vi "TachDataGcode_PosToQueue.vi"(8 "error in (no error)":errorcluster, 10 "outPOS":T1, 11 "Queue in":refnum<queue>) -> (0 "error out":errorcluster)   [LabVIEW 2017]
uses:
  controls/CommandQueue.ctl
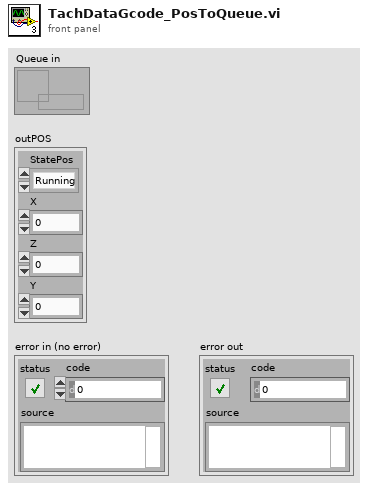
[diagram p1: front panel]
types:
  T1 = cluster{"StatePos":enum16{"Running", "Waiting", "Pos", "IDLE"}, "X":dbl, "Z":dbl, "Y":dbl}
  T2 = typedef "CommandQueue.ctl" = enum16{"updatePos", "UpdateConfigAccel", "UpdateConfigFeed", "UpdateConfigUnit"}
  T3 = cluster{"Command":T2, cluster{"X":dbl, "Z":dbl, "Y":dbl}}
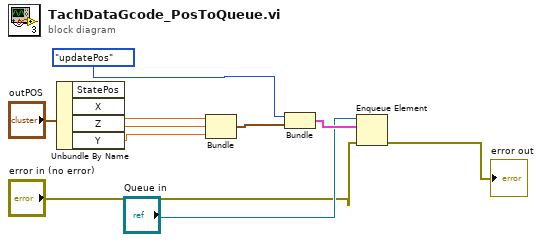
[diagram p0: block diagram]
diagram:
  n1 = Unbundle By Name("outPOS") -> ("X"=w1:dbl, "Z"=w6:dbl, "Y"=w2:dbl)  [unwired: 1 out]
  n2 = Bundle("X"=w1, "Z"=w6, "Y"=w2) -> (w7:cluster{"X":dbl, "Z":dbl, "Y":dbl})  [unwired: 1 in]
  n3 = Bundle("Command"=CommandQueue."updatePos", w7) -> (w10:T3)  [unwired: 1 in]
  n4 = Enqueue Element(queue="Queue in", element=w10, error in (no error)="error in (no error)") -> (error out=→"error out":errorcluster)  [unwired: 1 in, 2 out]
